vi "Channel 0 First Half (SubVI).vi"(0 "VISA Refnum in":refnum<visa-resource-name>, 1 "Channel #":i32, 2 "dt (s)":i32, 3 "Barcodes in":string[](array[string]), 8 "N":i32) -> (10 "Actual Voltage Level (V)":dbl format="%#_13g", 12 "OVV?":bool=TRUE, 14 "Power Supply Trip":bool, 16 "OVC?":bool=TRUE, 17 "Boolean 2":bool, 18 "Actual Current Limit (nA)":dbl format="%#_13g", 19 "BoardHandle out 2":T1, 20 "VISA Refnum out":refnum<visa-resource-name>, 21 "Time Left (s)":dbl, 22 "Manual Measurments \nNeeded":bool, 23 "Barcodes out":string[](array[string]), 24 "Boolean":bool, 25 "Channel # out 2":i32, 26 "Array":dbl[](array[numeric]), 27 "error out":errorcluster)   [LabVIEW 2020]
uses:
  <instrlib>/CAEN PSM/CAEN PSM.lvlib
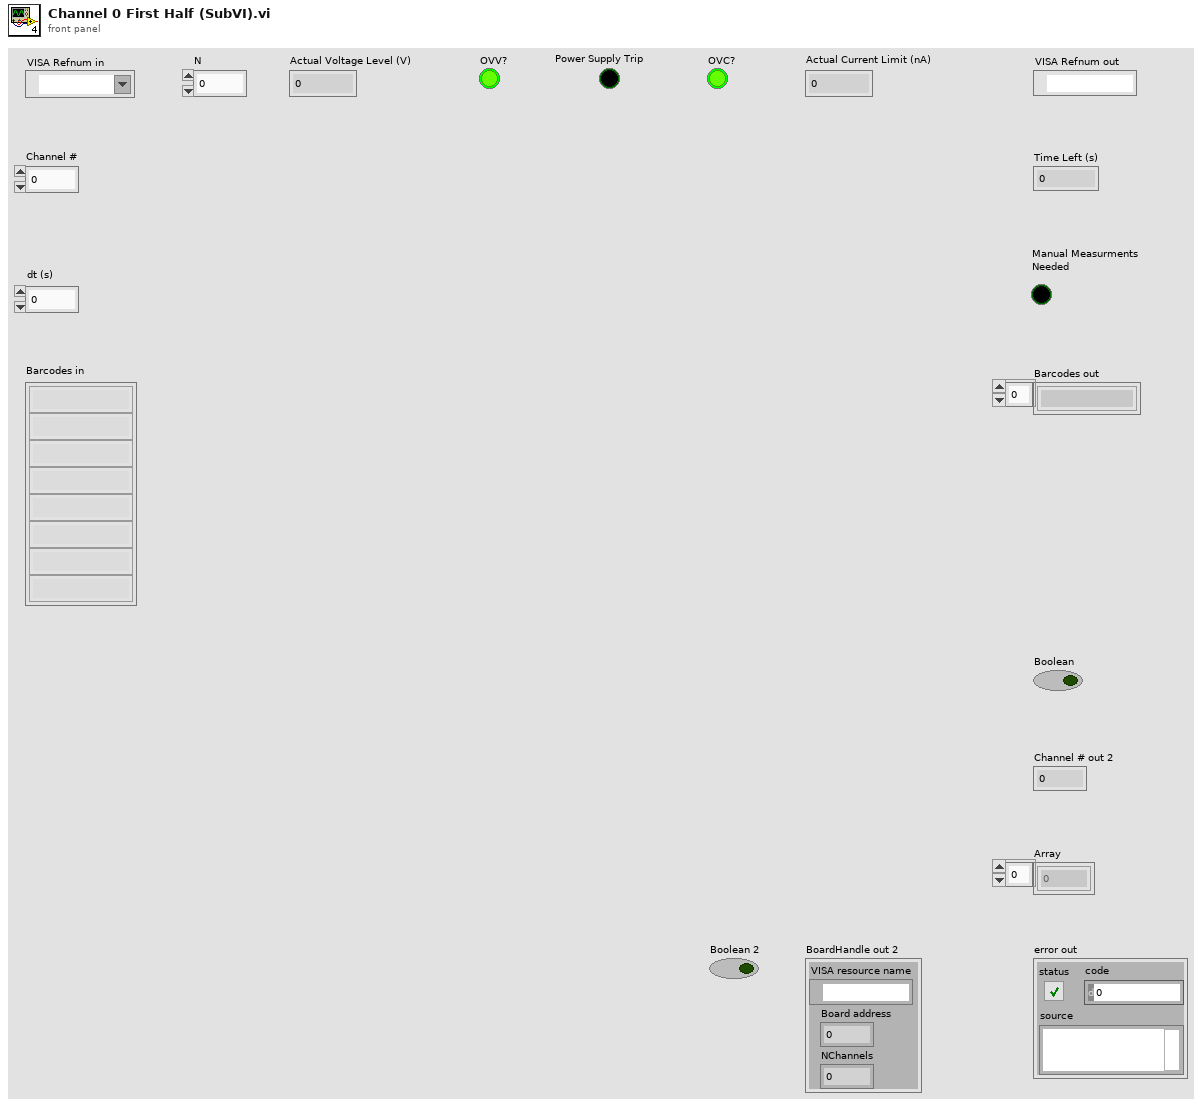
[diagram p1: front panel]
types:
  T1 = cluster{"VISA resource name":refnum<visa-resource-name>, "Board address":u8, "NChannels":u8}
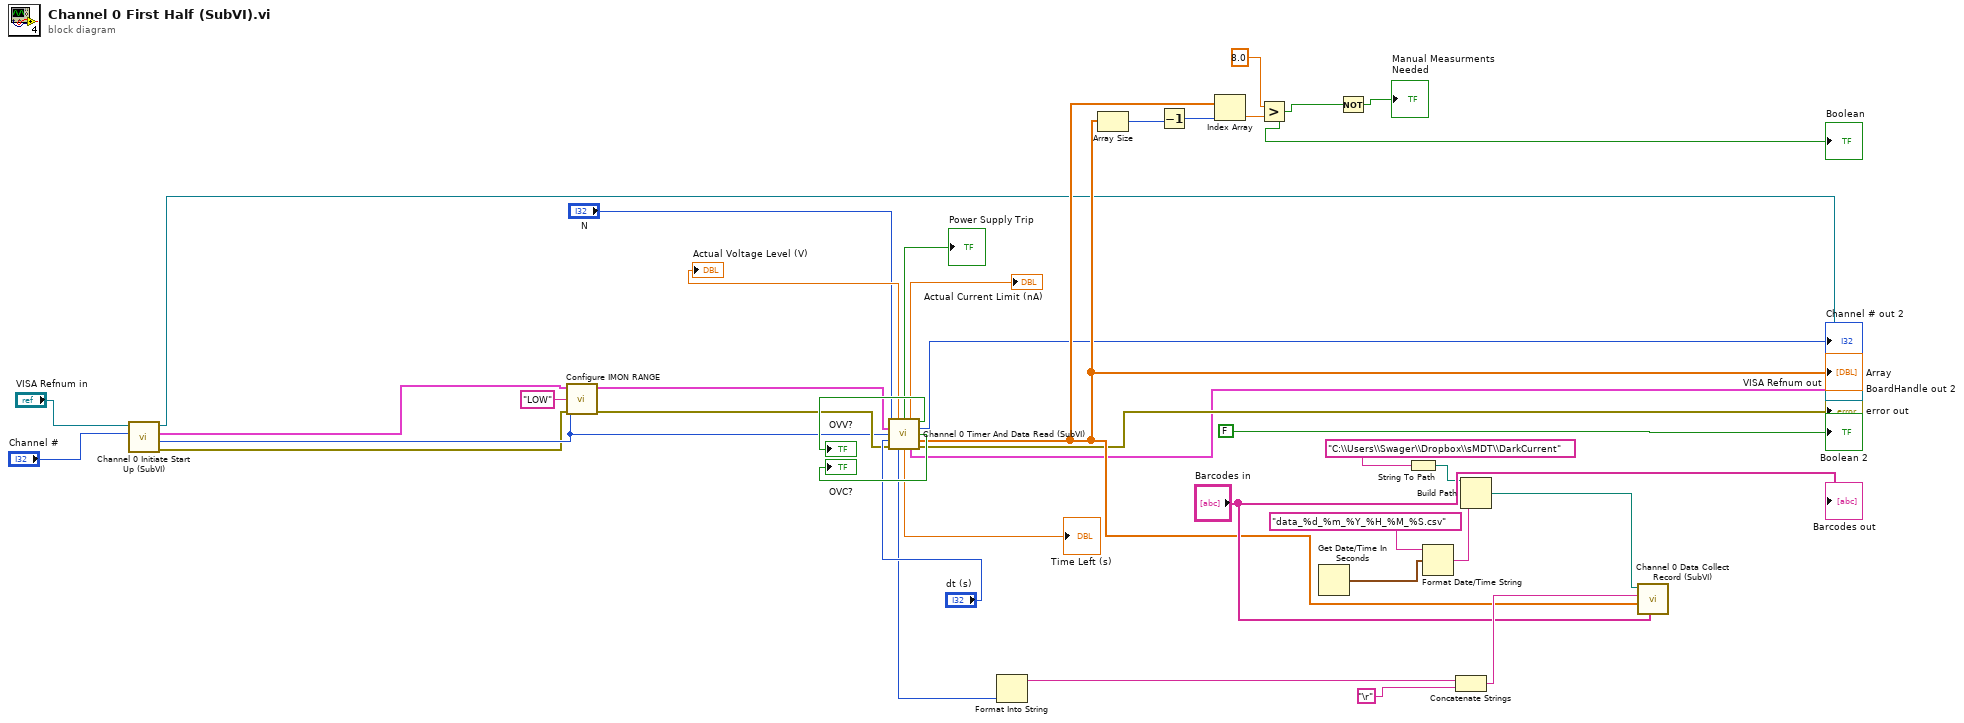
[diagram p0: block diagram]
diagram:
  n1 = call "Channel 0 Initiate Start Up (SubVI).vi"("Channel # in"="Channel #", "VISA Refnum in"="VISA Refnum in") -> ("error out"=w8:errorcluster, "Channel # out"=w11:i32, "BoardHandle out"=w9:T1, "VISA Refnum out"=→"VISA Refnum out":refnum<visa-resource-name>)  [unwired: 6 in]
  n2 = call <instrlib>:"Configure IMON RANGE.vi"("error in (no error)"=w8, "IMon range (LOW)"="LOW", "Channel (0)"=w11, "BoardHandle"=w9) -> ("error out"=w13:errorcluster, "BoardHandle out"=w12:T1)  [unwired: 6 in]
  n3 = call "Channel 0 Timer And Data Read (SubVI).vi"("N"="N", "BoardHandle in"=w12, "Channel # in"=w11, "dt (s) in"="dt (s)", "error in (no error)"=w13) -> ("Actual Voltage Level (V)"=→"Actual Voltage Level (V)":dbl, "Power Supply Trip"=→"Power Supply Trip":bool, "Actual Current Limit (nA)"=→"Actual Current Limit (nA)":dbl, "OVV?"=→"OVV?":bool, "Channel # out 2"=→"Channel # out 2":i32, "OVC?"=→"OVC?":bool, "Array"=w25:dbl[], "dt (s) out"=w26:i32, "Time Left (s)"=→"Time Left (s)":dbl, "BoardHandle out 2"=→"BoardHandle out 2":T1, "error out"=→"error out":errorcluster)
  "Array" <- w25
  n4 = Format Into String(w26) -> (resulting string=w30:string)  [unwired: 3 in, 1 out]
  n5 = Array Size(array=w25) -> (size(s)=w14:i32)
  n6 = Decrement(x=w14) -> (x-1=w15:i32)
  n7 = Index Array(array=w25, index=w15) -> (element=w16:dbl)
  n8 = Greater?(x=8.0, y=w16) -> (0:w17:bool)
  "Boolean" <- w17
  n9 = Get Date/Time In Seconds() -> (seconds since 1Jan1904=w22:timestamp)
  n10 = Not(x=w17) -> (.not. x?=→"Manual Measurments \nNeeded":bool)
  n11 = String To Path(string="C:\\Users\\Swager\\Dropbox\\sMDT\\DarkCurrent") -> (path=w23:path)
  n12 = Format Date/Time String(time format string (%c)="data_%d_%m_%Y_%H_%M_%S.csv", seconds (now)=w22) -> (date/time string=w21:string)  [unwired: 1 in]
  n13 = Concatenate Strings(w30, "\r") -> (w29:string)
  n14 = Build Path(base path=w23, name or relative path=w21) -> (appended path=w27:path)
  n15 = call "Channel 0 Data Collect Record (SubVI).vi"("Barcodes"="Barcodes in", "Array"=w25, "String"=w29, "appended path"=w27) -> ()  [unwired: 8 in]
  "Barcodes out" <- "Barcodes in"
  "Boolean 2" <- FALSE
